vi "add err msg to log.vi"(0 "Str Refnum":refnum<vi>, 5 "error in (no error)":errorcluster) -> ()   [LabVIEW 2014, in "PTUtils.lvlib"]
uses:
  PTUtils.lvlib
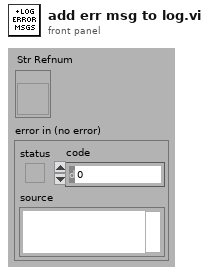
[diagram p1: front panel]
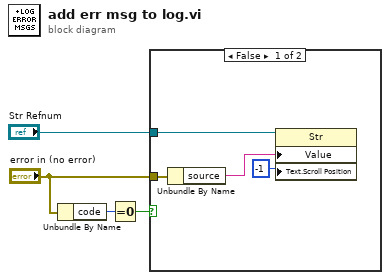
[diagram p0: block diagram]
diagram:
  n1 = Unbundle By Name("error in (no error)") -> ("code"=w3:i32)
  n2 = Equal To 0?(x=w3) -> (x = 0?=w2:bool)
  n3 = case shown="False" w2 {
    tunnel: "Str Refnum" -> [w6 _]
    tunnel: "error in (no error)" -> [w8 _]
    frame False {
      n4 = Unbundle By Name(w8) -> ("source"=w5:string)
      n5 = property on="Property Node" class="Str"(reference=w6, "Value"=w5, "Text.Scroll Position"=-1) -> ()  [unwired: 1 in, 2 out]
    }
    frame True {
    }
  }
